vi "T7_Read_Single.vi"(8 "error in (no error)":errorcluster, 9 "Starting Address":u16, 10 "Remote Port":u16=502, 11 "Remote IP Address":string="192.168.1.15") -> (0 "error out":errorcluster, 2 "Value":sgl)   [LabVIEW 2013]
uses:
  Serial Link Layer/NI_Modbus_Cleaned/NI Modbus121Clean.llb/MB Ethernet Master Query Read Input Registers (poly).vi
panel:
  in  "Num Registers":u16=2
  out "Array":sgl[](array[numeric])
  out "Results (binary)":u16[](array[numeric])
  # "TCP Parameters"
  # "Slave Read-only Registers"
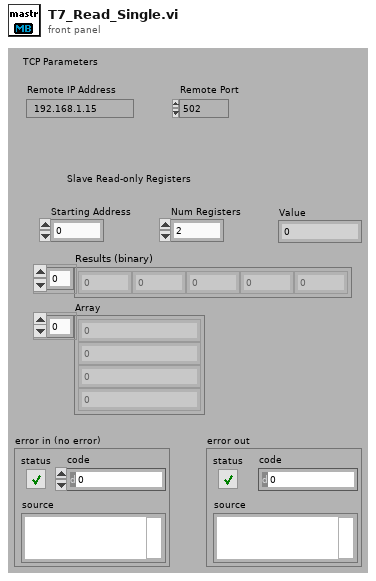
[diagram p1: front panel]
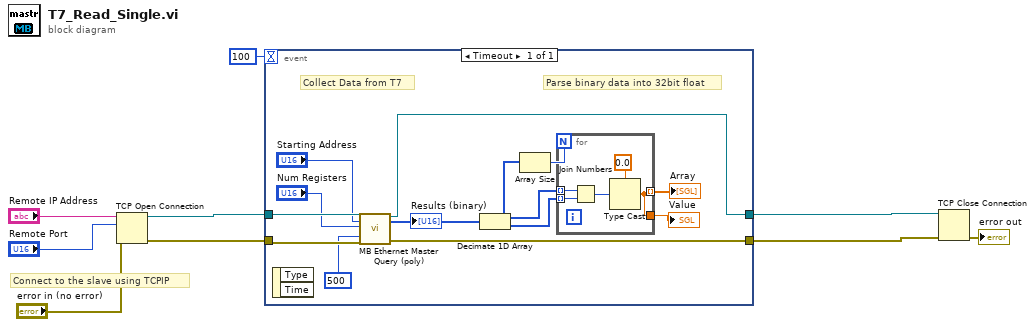
[diagram p0: block diagram]
diagram:
  # "Connect to the slave using TCPIP"
  n1 = TCP Open Connection(address="Remote IP Address", remote port or service name="Remote Port", error in (no error)="error in (no error)") -> (connection ID=w7:refnum<k5>, error out=w6:errorcluster)  [unwired: 2 in]
  n2 = event shown="[0] Timeout" {
    selector: _ -> [_]
    dyn-events: _ -> [_]
    timeout: 100 -> [_]
    tunnel: [w17] -> w5
    tunnel: w7 -> [w22]
    tunnel: w6 -> [w20]
    tunnel: [w18] -> w4
    event Timeout {
      # "Parse binary data into 32bit float"
      # "Collect Data from T7"
      n3 = event-data() -> ()  [unwired: 3 out]
      n4 = call-poly "MB Ethernet Master Query (poly).vi"("TCP Connection Refnum in"=w22, "Starting Address"="Starting Address", "Quantity"="Num Registers", "Timeout"=500, "error in"=w20) -> ("TCP Connection Refnum (dup)"=w18:refnum<k5>, "Input Registers"=w16:u16[], "error out"=w17:errorcluster)  [unwired: 11 in, 1 out]
      "Results (binary)" <- w16
      n5 = Decimate 1D Array(w16) -> (w14:u16[], w13:u16[])
      n6 = Array Size(array=w14) -> (size(s)=w15:i32)
      n7 = for {
        N: w15 -> [_]
        tunnel: w14 -> [w26] mode=indexing
        tunnel: w13 -> [w27] mode=indexing
        tunnel: [w23] -> w12 mode=indexing
        tunnel: [w23] -> w11
        n8 = Join Numbers(hi=w26, lo=w27) -> ((hi.lo)=w25:u32)
        n9 = Type Cast(type=sgl 0.0, x=w25) -> (*(type *) &x=w23:sgl)
      }
      "Array" <- w12
      "Value" <- w11
    }
  }
  n10 = TCP Close Connection(connection ID=w4, error in (no error)=w5) -> (error out=→"error out":errorcluster)  [unwired: 2 out]
